vi "RTS Send File Setup Data.vi"(8 "Error In":errorcluster, 9 "Setup Info":string, 10 "Tree Selection":T1, 11 "path":path) -> (0 "Error Out":errorcluster, 3 "File Setup Data":string)   [LabVIEW 2020]
uses:
  Type Definitions/RTS Room Selector.ctl
  Type Definitions/RTS TCP Commands.ctl
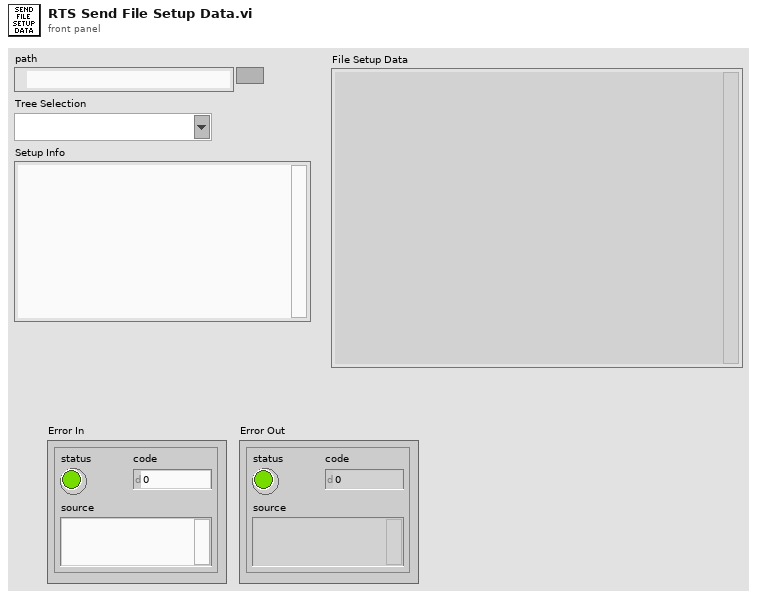
[diagram p1: front panel]
types:
  T1 = typedef "RTS Room Selector.ctl" = string
  T2 = typedef "RTS TCP Commands.ctl" = string
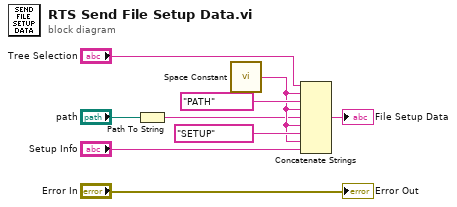
[diagram p0: block diagram]
diagram:
  n1 = Path To String(path="path") -> (string=w5:string)
  n2 = call <vilib>:"Space Constant.vi"() -> ("String"=w6:string)
  n3 = Concatenate Strings("Tree Selection", w6, T2 "PATH" ("TCP Commands"), w6, w5, w6, T2 "SETUP" ("TCP Commands"), w6, "Setup Info") -> (→"File Setup Data":string)
  "Error Out" <- "Error In"
